vi "ConfigureExposureTime.vi"(0 "object in":refnum<class "Hamamatsu.lvclass">, 2 "ExposureTime(ms)":dbl, 5 "error in (no error)":errorcluster) -> (14 "object out":refnum<class "Hamamatsu.lvclass">, 19 "error out":errorcluster)   [LabVIEW 2021, in "Hamamatsu.lvclass"]
uses:
  Hamamatsu.lvclass
  Hamamatsu.lvclass/Hamamatsu.ctl
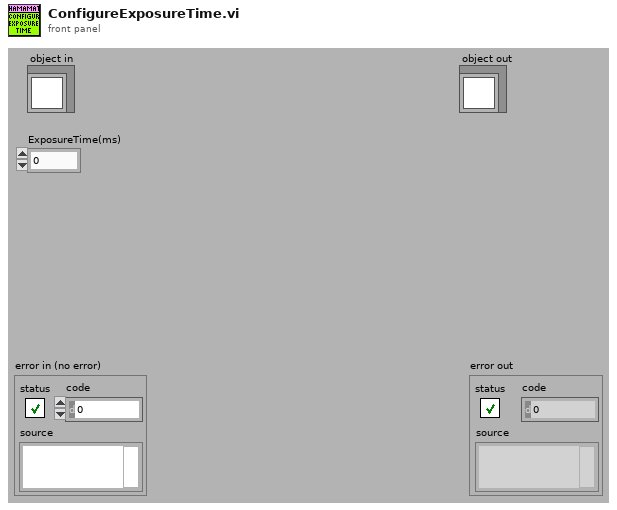
[diagram p1: front panel]
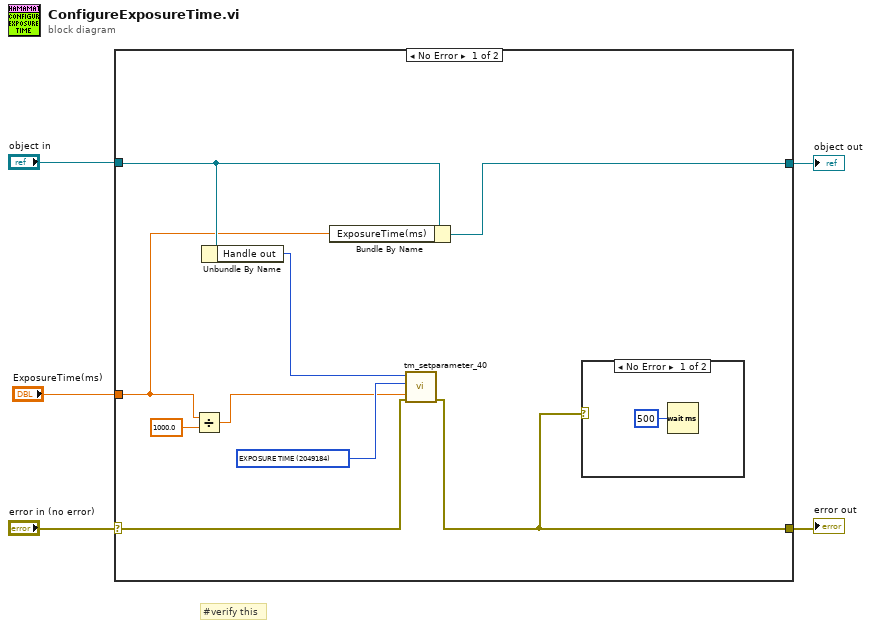
[diagram p0: block diagram]
diagram:
  # "#verify this"
  n1 = case shown="No Error" "error in (no error)" {
    selector: "error in (no error)" -> [w12 w17]
    tunnel: [w11 w17] -> w4
    tunnel: [w8 w16] -> w2
    tunnel: "object in" -> [w7 w16]
    tunnel: "ExposureTime(ms)" -> [w6 _]
    frame No Error {
      w13 = u32 2049184 items=["SENSOR MODE"=4212128, "SENSOR MODE LINE BUNDLE HEIGHT"=4212192, "READOUT DIRECTION"=4211904, "BIT PER CHANNEL"=4342976, "EXPOSURE TIME"=2049184, "CONTRAST GAIN"=3163312, "BINNING"=4215968, "TIMING READOUT TIME"=4223904, "INTERNAL FRAME RATE"=4225952, "INTERNAL FRAME INTERVAL"=4225968, "INTERNAL LINE SPEED"=4226000, "IMAGE WIDTH"=4343200, "IMAGE HEIGHT"=4343216, "IMAGE ROWBYTES"=4343232, "IMAGE FRAMEBYTES"=4343248, "IMAGE PIXEL TYPE"=4343296] ("Parameter")
      n2 = Divide(x=w6, y=1000.0) -> (x/y=w10:dbl)
      n3 = Unbundle By Name(w7) -> ("Handle out"=w14:u32)
      n4 = Bundle By Name(cluster=w7, "ExposureTime(ms)"=w6) -> (w8:refnum<class "Hamamatsu.lvclass">)
      n5 = call <userlib>:"tm_setparameter_40.vi"("error in (no error)"=w12, "Value in"=w10, "Parameter"=w13, "Handle in"=w14) -> ("error out"=w11:errorcluster)  [unwired: 6 in, 1 out]
      n6 = case shown="No Error" w11 {
        frame No Error {
          n7 = Wait (ms)(milliseconds to wait=u32 500) -> ()  [unwired: 1 out]
        }
        frame Error {
        }
      }
    }
    frame Error {
    }
  }
  "error out" <- w4
  "object out" <- w2
